vi "alinha-com-parede.vi"(4 "NXT/EV3":T1) -> (1 "NXT/EV3 2":T1)   [LabVIEW 2016]
uses:
  <vilib>/NXT/Subs/LVHSConnector.ctl
  <vilib>/NXT/LegoClasses/BrickReference/BrickReference.lvclass
  <vilib>/NXT/Block Support/NXT_OutputPort.ctl
  <vilib>/NXT/Block Support/NXT_InputPort.ctl
  <vilib>/NXT/Dual Mode Library/Motors/ResetMotor.vi
  <vilib>/NXT/Dual Mode Library/Sensors/Touch_Pressed.vi
  <vilib>/NXT/NXTIO Xnodes/NXTIONodeSubVIs/NXTMoveMotors.vi
  <vilib>/NXT/Dual Mode Library/Motors/Rotation.vi
  <vilib>/NXT/NXTIO Xnodes/AddressXNode/NXTIOAddress.xnode
  <vilib>/NXT/NXTIO Xnodes/NXTIOXNode/NXTIO.xnode
panel:
  out "Angle of Rotation":i32
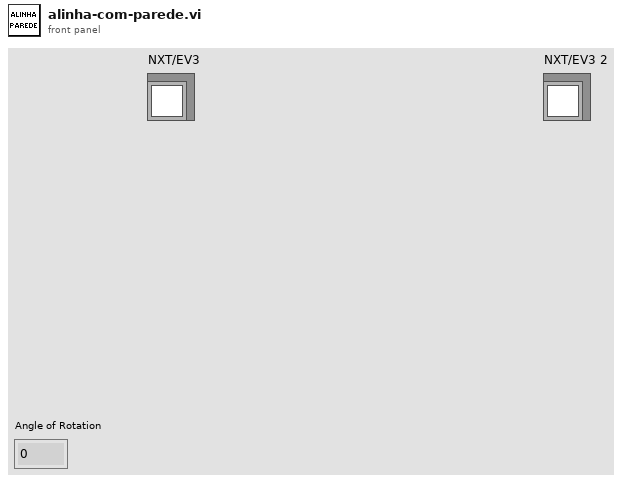
[diagram p1: front panel]
types:
  T1 = typedef "LVHSConnector.ctl" = refnum<class "BrickReference.lvclass">
  T2 = typedef "NXT_OutputPort.ctl" = u8
  T3 = typedef "NXT_InputPort.ctl" = u32
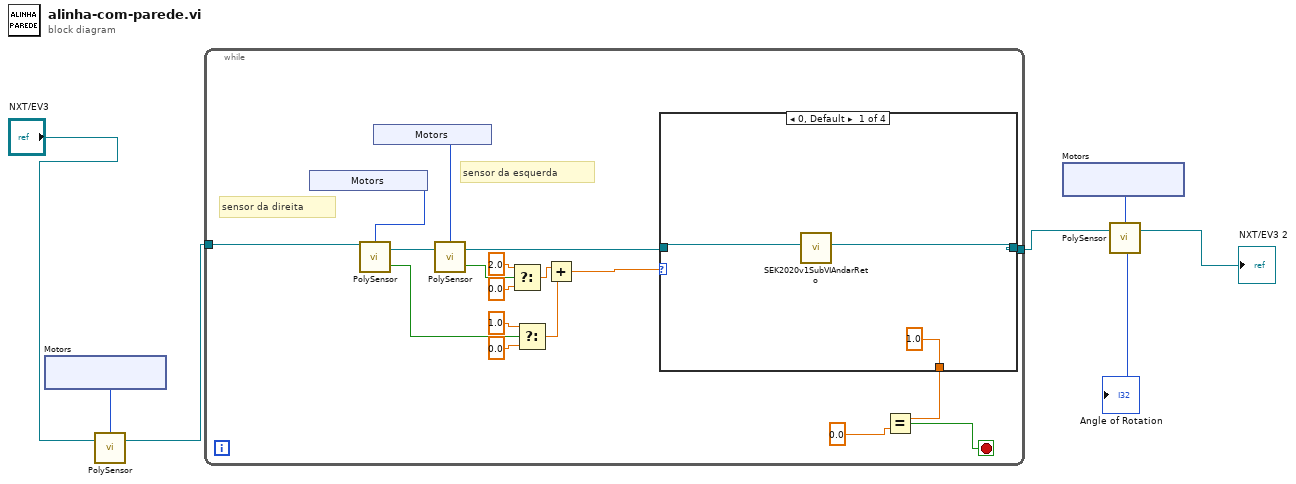
[diagram p0: block diagram]
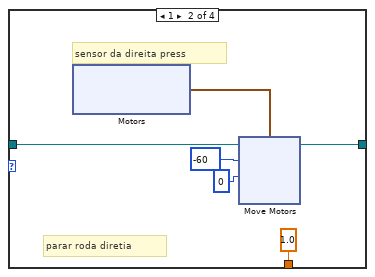
[diagram p2: hidden frame]
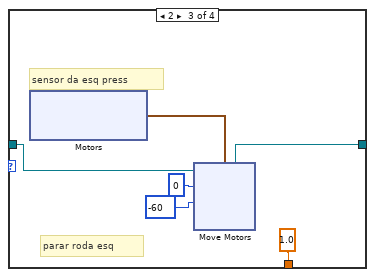
[diagram p3: hidden frame]
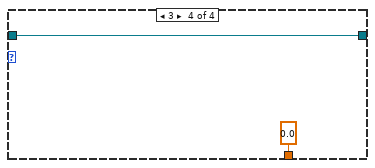
[diagram p4: hidden frame]
diagram:
  n1 = xnode "Motors"() -> ("Motor"=w7:T2)
  n2 = call-poly <vilib>:"PolySensor.vi"("NXT/EV3"="NXT/EV3", "Port (All Ports)"=w7) -> ("NXT/EV3"=w1:T1)  [unwired: 2 out]
  n3 = while {
    tunnel: w1 -> [w8]
    tunnel: [w18] -> w4
    stop <- w15 stop-if-true
    # "sensor da esquerda"
    # "sensor da direita"
    n4 = xnode "Motors"() -> ("Sensor"=w14:T3)
    n5 = call-poly <vilib>:"PolySensor.vi"("NXT/EV3"=w8, "Port (Port 1)"=w14) -> ("Yes / No"=w24:bool, "NXT/EV3"=w25:T1)  [unwired: 1 in]
    n6 = xnode "Motors"() -> ("Sensor"=w13:T3)
    n7 = call-poly <vilib>:"PolySensor.vi"("NXT/EV3"=w25, "Port (Port 1)"=w13) -> ("Yes / No"=w19:bool, "NXT/EV3"=w9:T1)  [unwired: 1 in]
    n8 = Select(t=2.0, s=w19, f=0.0 ("t")) -> (s? t:f=w12:dbl)
    n9 = Select(t=1.0, s=w24, f=0.0 ("t")) -> (s? t:f=w11:dbl)
    n10 = Add(x=w12, y=w11) -> (x+y=w10:dbl)
    n11 = case shown="0, Default" w10 {
      tunnel: w9 -> [w29 w33 w48 w62]
      tunnel: [w30 w32 w47 w62] -> w18
      tunnel: [1.0 ("t") 1.0 ("t") 1.0 ("t") 0.0 ("t")] -> w17
      frame 0, Default {
        n12 = call "SEK2020v1SubVIAndarReto.vi"("NXT/EV3"=w29) -> ("NXT/EV3 2"=w30:T1)  [unwired: 9 in]
      }
      frame 1 {
        # "parar roda diretia"
        # "sensor da direita press"
        n13 = xnode "Motors"() -> ("Motor"=w34:cluster{"Port":T2, "Port":T2})
        n14 = xnode "Move Motors"("Power/Speed 2"=i8 0, "Power/Speed 1"=i8 -60, "Motors"=w34, "NXT/EV3"=w33) -> ("NXT/EV3"=w32:T1)
      }
      frame 2 {
        # "parar roda esq"
        # "sensor da esq press"
        n15 = xnode "Motors"() -> ("Motor"=w51:cluster{"Port":T2, "Port":T2})
        n16 = xnode "Move Motors"("Power/Speed 2"=i8 -60 ("Power/Speed 1"), "Power/Speed 1"=i8 0 ("Power/Speed 2"), "Motors"=w51, "NXT/EV3"=w48) -> ("NXT/EV3"=w47:T1)
      }
      frame 3 {
      }
    }
    n17 = Equal?(x=w17, y=0.0 ("t")) -> (x = y?=w15:bool)
  }
  n18 = xnode "Motors"() -> ("Motor"=w6:T2)
  n19 = call-poly <vilib>:"PolySensor.vi"("NXT/EV3"=w4, "Port (Port A)"=w6) -> ("Angle of Rotation"=→"Angle of Rotation":i32, "NXT/EV3"=→"NXT/EV3 2":T1)  [unwired: 1 out]
